vi "Create PPL.vi"(0 "Project Refnum":refnum<vi>, 5 "Plug-in name":string, 11 "error in (no error)":errorcluster) -> (4 "project ref out":refnum<vi>, 15 "error out":errorcluster)   [LabVIEW 2021, in "NI_AB_API_PPL_Extensions.lvclass"]
uses:
  NI_AB_API_PPL_Extensions.lvclass
  NI_AB_API_PPL_Extensions.lvclass/NI_AB_API_PPL_Extensions.ctl
  InstrumentStudio Plug-In Editor.lvlib
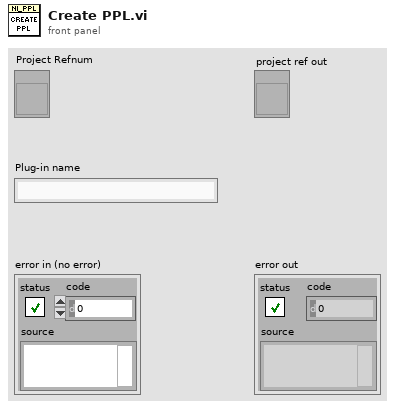
[diagram p1: front panel]
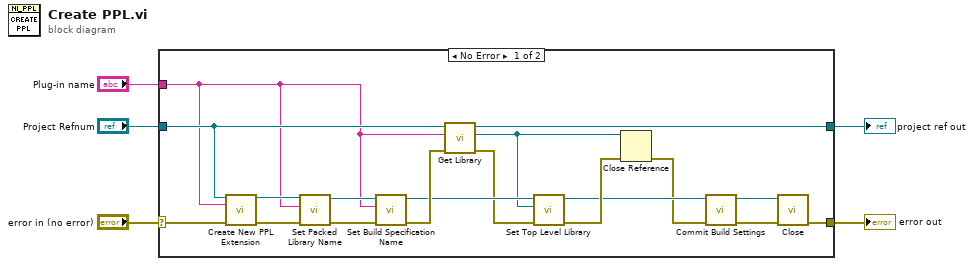
[diagram p0: block diagram]
diagram:
  n1 = case shown="No Error" "error in (no error)" {
    selector: "error in (no error)" -> [w23 w25]
    tunnel: [w9 w25] -> w2
    tunnel: "Project Refnum" -> [w22 w24]
    tunnel: "Plug-in name" -> [w6 _]
    tunnel: [w11 w24] -> w3
    frame No Error {
      n2 = call "Create New PPL Extension.vi"("Project Refnum"=w22, "Build specification name"=w6, "error in (no error)"=w23) -> ("NI_AB_API_Build out"=w15:refnum<class "NI_AB_API_PPL_Extensions.lvclass">, "error out"=w12:errorcluster)  [unwired: 11 in]
      n3 = call-dynamic "Set Packed Library Name.vi"("error in (no error)"=w12, "Packed library name"=w6, "PPL in"=w15) -> ("error out"=w13:errorcluster, "PPL out"=w14:refnum<class "NI_AB_API_PPL_Extensions.lvclass">)  [unwired: 7 in]
      n4 = call-dynamic "Set Build Specification Name.vi"("error in (no error)"=w13, "Build Specification Name"=w6, "NI_AB_API_PPL in"=w14) -> ("error out"=w21:errorcluster, "NI_AB_API_PPL out"=w20:refnum<class "NI_AB_API_PPL_Extensions.lvclass">)  [unwired: 7 in]
      n5 = call "Get Library.vi"("error in"=w21, "library name"=w6, "project ref"=w22) -> ("error out"=w19:errorcluster, "library item"=w8:refnum<vi>, "project ref out"=w11:refnum<vi>)  [unwired: 5 in, 1 out]
      n6 = call-dynamic "Set Top Level Library.vi"("error in (no error)"=w19, "ProjectItem Refnum"=w8, "PPL in"=w20) -> ("error out"=w17:errorcluster, "PPL out"=w10:refnum<class "NI_AB_API_PPL_Extensions.lvclass">)  [unwired: 7 in]
      n7 = Close Reference(reference=w8, error in (no error)=w17) -> (error out=w7:errorcluster)
      n8 = call-dynamic "Commit Build Settings.vi"("error in (no error)"=w7, "PPL in"=w10) -> ("error out"=w18:errorcluster, "PPL out"=w16:refnum<class "NI_AB_API_PPL_Extensions.lvclass">)  [unwired: 8 in]
      n9 = call-dynamic "Close.vi"("error in (no error)"=w18, "DLL in"=w16) -> ("error out"=w9:errorcluster)  [unwired: 9 in]
    }
    frame Error {
    }
  }
  "error out" <- w2
  "project ref out" <- w3
